vi "PostCopyScripting.vi"(10 "MetaDataObj":refnum<class "MetaDataObj.lvclass">, 11 "User Project":refnum<vi>) -> ()   [LabVIEW 2020, in "CCMazeMetaDataObj.lvclass"]
uses:
  CCMazeMetaDataObj.lvclass
  <resource>/dialog/NewProjectWizard/MetaDataObj/MetaDataObj.lvclass
  <vilib>/AppBuilder/AB_API/PPL/NI_AB_API_PPL.lvclass
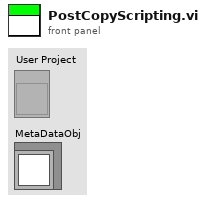
[diagram p1: front panel]
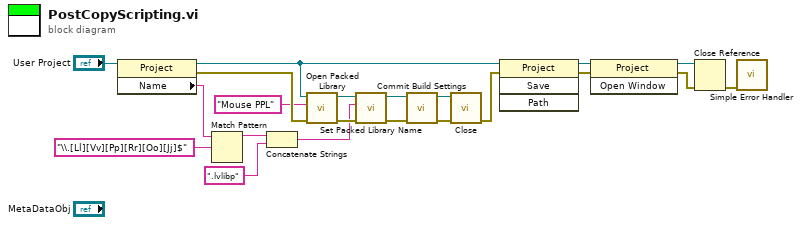
[diagram p0: block diagram]
diagram:
  n1 = property class="Project"(reference="User Project") -> (reference out=w5:refnum<vi>, error out=w21:errorcluster, "Name"=w19:string)  [unwired: 1 in]
  n2 = Match Pattern(string=w19, regular expression="\\.[Ll][Vv][Pp][Rr][Oo][Jj]$") -> (before substring=w14:string)  [unwired: 1 in, 3 out]
  n3 = Concatenate Strings(w14, ".lvlibp" ("string")) -> (w12:string)
  n4 = call <vilib>:"Open Packed Library.vi"("error in (no error)"=w21, "Build specification name"="Mouse PPL", "Project Refnum"=w5) -> ("error out"=w15:errorcluster, "PPL out"=w16:refnum<class "NI_AB_API_PPL.lvclass">)  [unwired: 7 in]
  n5 = call-dynamic "Set Packed Library Name.vi"("error in (no error)"=w15, "Packed library name"=w12, "PPL in"=w16) -> ("error out"=w10:errorcluster, "PPL out"=w11:refnum<class "NI_AB_API_PPL.lvclass">)  [unwired: 7 in]
  n6 = call-dynamic "Commit Build Settings.vi"("error in (no error)"=w10, "PPL in"=w11) -> ("error out"=w8:errorcluster, "PPL out"=w9:refnum<class "NI_AB_API_PPL.lvclass">)  [unwired: 8 in]
  n7 = call-dynamic "Close.vi"("error in (no error)"=w8, "DLL in"=w9) -> ("error out"=w4:errorcluster)  [unwired: 9 in]
  n8 = invoke class="Project" method="Save"(reference=w5, error in=w4) -> (reference out=w7:refnum<vi>, error out=w6:errorcluster)  [unwired: 2 in, 2 out]
  n9 = invoke class="Project" method="Open Window"(reference=w7, error in=w6) -> (reference out=w2:refnum<vi>, error out=w3:errorcluster)  [unwired: 1 in, 1 out]
  n10 = Close Reference(reference=w2, error in (no error)=w3) -> (error out=w1:errorcluster)
  n11 = call <vilib>:"Simple Error Handler.vi"("error in (no error)"=w1) -> ()  [unwired: 4 in, 5 out]
